vi "N-Channel 1-Sample (1D DBL).vi"() -> ()   [LabVIEW 2019]
uses:
  <vilib>/DAQmx/read.llb/DAQmx Read (Analog 1D DBL NChan 1Samp).vi
  <vilib>/DAQmx/create/channels.llb/DAQmx Create Channel (AI-Voltage-Basic).vi
  <vilib>/DAQmx/configure/timing.llb/DAQmx Timing (Sample Clock).vi
  <vilib>/DAQmx/miscellaneous.llb/DAQmx Fill In Error Info.vi
panel:
  out "1D Numeric Output":dbl[](array[numeric])
  out "Waveform Chart":T1(graph)
  in  "Stop":bool
  in  "Physical Channel":tag="PCI-6221/ai0, PCI-6221/ai2:3"
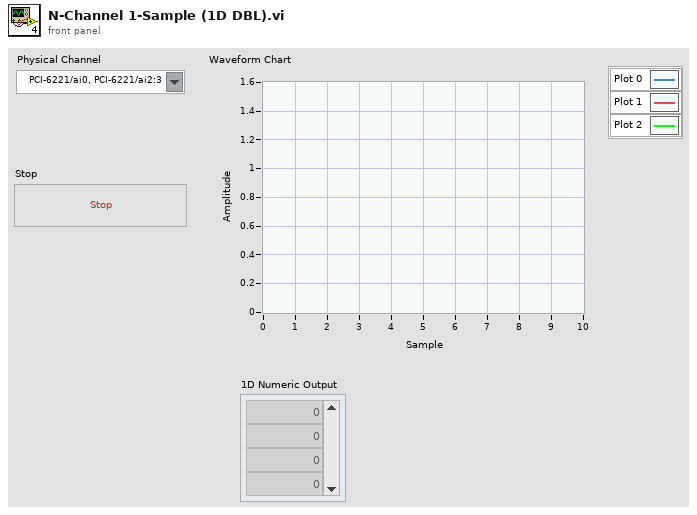
[diagram p1: front panel]
types:
  T1 = cluster{"data[0]":dbl, "data[1]":dbl, "data[2]":dbl, "data[3]":dbl, "data[4]":dbl, "data[5]":dbl, "data[6]":dbl, "data[7]":dbl, "data[8]":dbl}
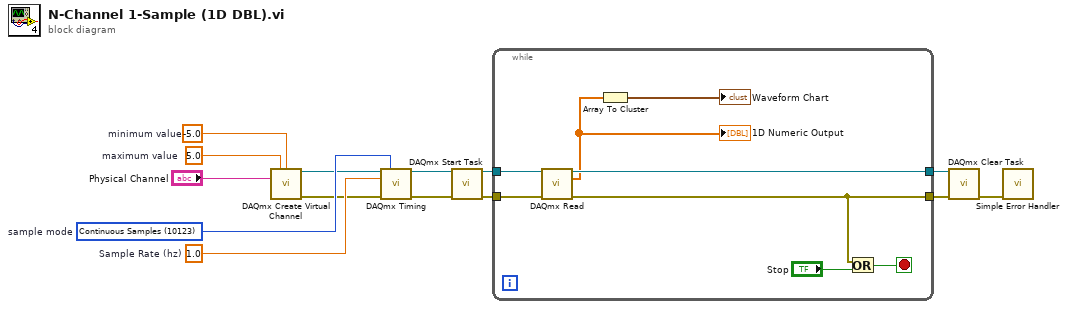
[diagram p0: block diagram]
diagram:
  w6 = 5.0  # maximum value
  w7 = -5.0  # minimum value
  w13 = 1.0  # Sample Rate (hz)
  w14 = 10123 items=["Finite Samples"=10178, "Continuous Samples"=10123, "Hardware Timed Single Point"=12522]  # sample mode
  n1 = call-poly <vilib>:"DAQmx Create Virtual Channel.vi"("maximum value"=w6, "minimum value"=w7, "physical channels"="Physical Channel") -> ("task out"=w12:refnum<k21>, "error out"=w11:errorcluster)  [unwired: 11 in]
  n2 = call-poly <vilib>:"DAQmx Timing.vi"("task/channels in"=w12, "sample mode"=w14, "rate"=w13, "error in"=w11) -> ("task out"=w10:refnum<k21>, "error out"=w9:errorcluster)  [unwired: 10 in]
  n3 = call <vilib>:"DAQmx Start Task.vi"("task/channels in"=w10, "error in"=w9) -> ("task out"=w2:refnum<k21>, "error out"=w1:errorcluster)  [unwired: 12 in]
  n4 = while {
    tunnel: [w22] -> w5
    tunnel: [w21] -> w4
    tunnel: w2 -> [w18]
    tunnel: w1 -> [w17]
    stop <- w19 stop-if-true
    n5 = call-poly <vilib>:"DAQmx Read.vi"("task/channels in"=w18, "error in"=w17) -> ("task out"=w22:refnum<k21>, "data"=w15:dbl[], "error out"=w21:errorcluster)  [unwired: 11 in]
    "1D Numeric Output" <- w15
    n6 = Array To Cluster(array=w15) -> (cluster=→"Waveform Chart":T1)
    n7 = Or(x=w21, y="Stop") -> (x .or. y?=w19:bool)
  }
  n8 = call <vilib>:"DAQmx Clear Task.vi"("task in"=w5, "error in"=w4) -> ("error out"=w3:errorcluster)  [unwired: 13 in]
  n9 = call <vilib>:"Simple Error Handler.vi"("error in (no error)"=w3) -> ()  [unwired: 4 in, 5 out]
